vi "eID_Image_Path.vi"() -> (3 "Path out":path)   [LabVIEW 2020]
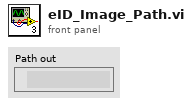
[diagram p1: front panel]
types:
  T1 = cluster{"Data Path":path, "Calibration Path":path, "Settings Path":path, "Script Path":path, "DAQ Support":path, "Reporting Desktop":path, "Help":path}
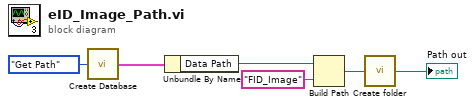
[diagram p0: block diagram]
diagram:
  n1 = call <userlib>:"Create Database.vi"("Get/Create"=enum16{"Get Path", "Create Path"}."Get Path") -> ("Path Out"=w2:T1)  [unwired: 13 in, 1 out]
  n2 = Unbundle By Name(w2) -> ("Data Path"=w3:path)
  n3 = Build Path(base path=w3, name or relative path="FID_Image") -> (appended path=w5:path)
  n4 = call <userlib>:"Create folder.vi"("Path In"=w5) -> ("Path out"=→"Path out":path)  [unwired: 14 in]
